vi "AutoCAD cmds testing.vi"(6 "AutoCAD cmd":T3, 7 "MathCAD results":T2, 8 "error in (no error)":errorcluster, 9 "path":path=path "C:/Documents and Settings/mw24/My Documents/Drawing2.dwg", 10 "Command":string="box 4 4 4\n_-view\n_swiso\n_shademode\nRealistic ") -> (0 "error out":errorcluster, 2 "IsQuiescent":bool)   [LabVIEW 2010]
uses:
  AutoCAD cmds.ctl
  MathCAD results ref.ctl
  Project commands.ctl
  AguaClara Library.lvlib
panel:
  in  "AcSaveAsType":T1(ring)
  out "new doc error":errorcluster
  out "Iterations":i32
  out "Visible":bool
  out "appended path":path
  out "basepath":string
  # "acR14_dwg\n AutoCAD R14 DWG (*.dwg)\n \nac2000_dwg\n AutoCAD 2000 DWG (*.dwg)\n \nac2000_dxf\n AutoCAD 2000 DXF (*.dxf)\n \nac2000_Template\n AutoCAD 2000 Drawing Template File (*.dwt)\n \nac2004_dwg\n AutoCAD 2004 DWG (*.dwg)\n \nac2004_dxf\n AutoCAD 2004 DXF (*.dxf)\n \nac2004_Template\n AutoCAD 2004 Drawing Template File (*.dwt)\n \nac2007_dwg\n AutoCAD 2007 DWG (*.dwg)\n \nac2007_dxf\n AutoCAD 2007 DXF (*.dxf)\n \nac2007_Template\n AutoCAD 2007 Drawing Template File (*.dwt)\n \nacNative\n A synonym for the latest drawing release. In this release, this value equals ac2007_dwg."
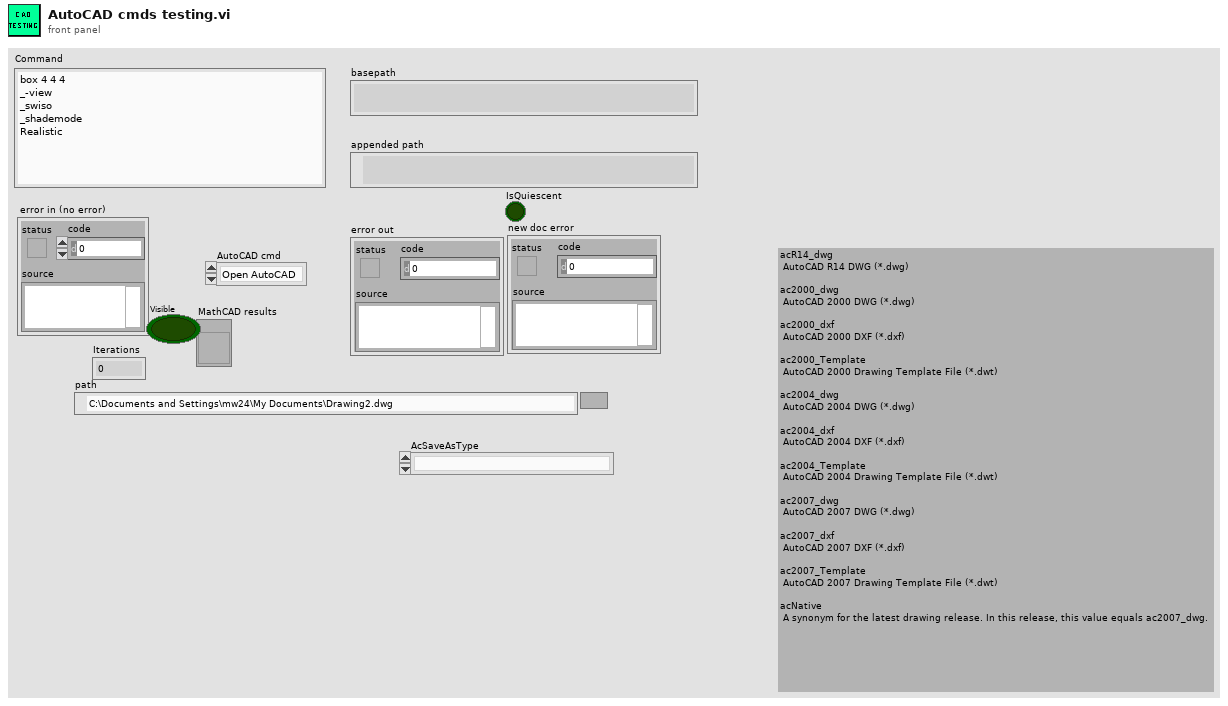
[diagram p1: front panel]
types:
  T1 = enum16{"", "acR14_dwg", "ac2000_dwg", "ac2000_dxf", "ac2000_Template", "ac2004_dwg", "ac2004_dxf", "ac2004_Template", "ac2007_dwg", "ac2007_dxf", "ac2007_Template", "acNative"}
  T2 = typedef "MathCAD results ref.ctl" = refnum<vi>
  T3 = typedef "AguaClara Library.lvlib/AutoCAD cmds.ctl" = enum16{"Open AutoCAD", "New Document", "Send Command", "Send Command Array", "Save picture", "Save File", "Close Doc", "Quit"}
  T4 = typedef "AguaClara Library.lvlib/Project commands.ctl" = enum16{"Load base file", "Load User", "Read paths", "Open Project", "New project", "Edit project", "Delete project", "Mail project", "save design", "open design"}
  T5 = cluster{"Label.Text":string, "Caption.Text":string[], "Control Type":u32, "Numeric":dbl, "Array":dbl[], "status":bool, "Outputs":bool[], "Str Array":string[], "String":string}[]
  T6 = typedef "AguaClara Library.lvlib/File paths.ctl" = cluster{"basepath":string, "AutoCAD script":string, "Design variables":string}
  T7 = typedef "AguaClara Library.lvlib/Project inputs.ctl" = cluster{"Project Name":string, "City":string, "State":string, "Country":string, "Notes":string}
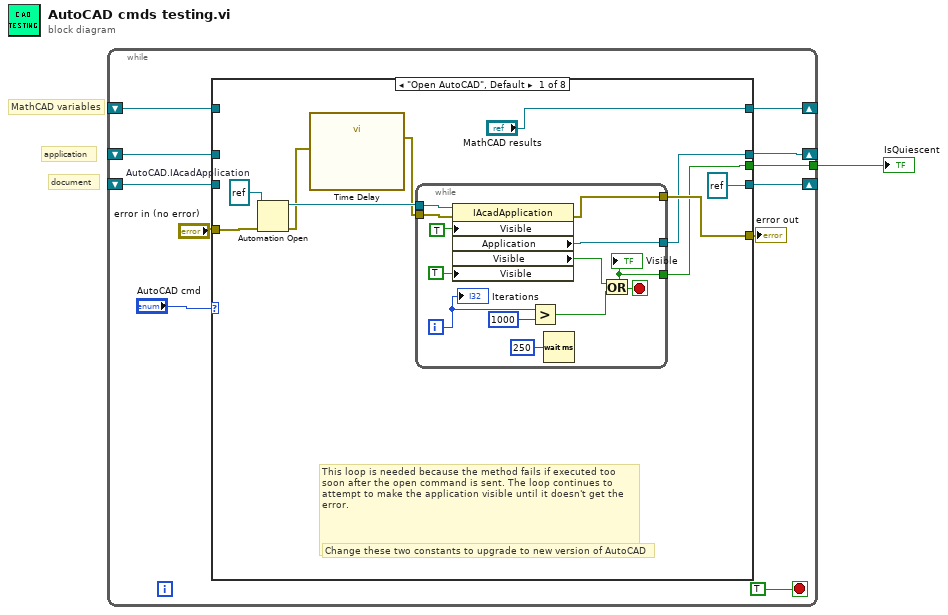
[diagram p0: block diagram]
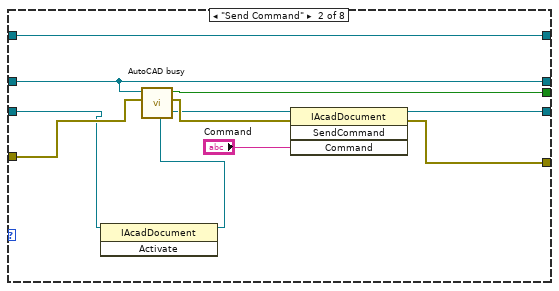
[diagram p2: hidden frame]
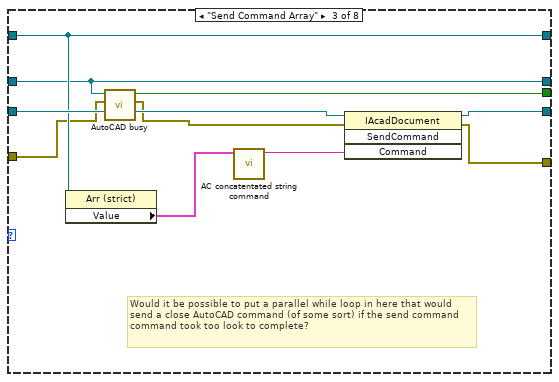
[diagram p3: hidden frame]
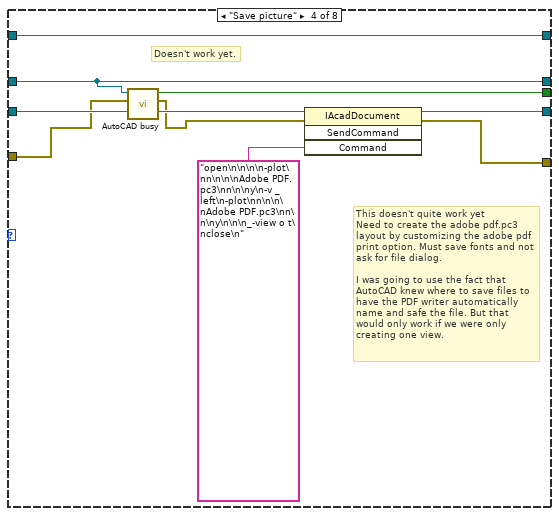
[diagram p4: hidden frame]
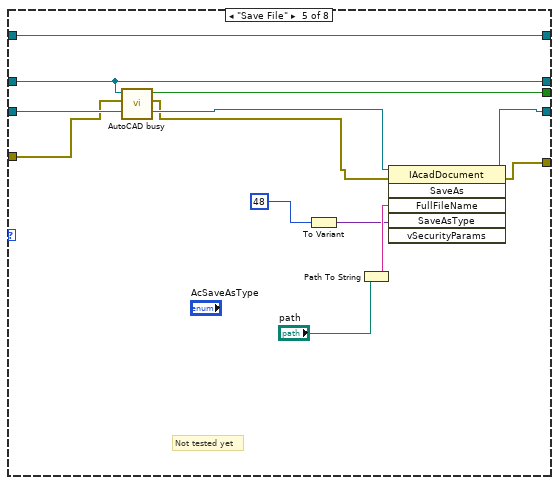
[diagram p5: hidden frame]
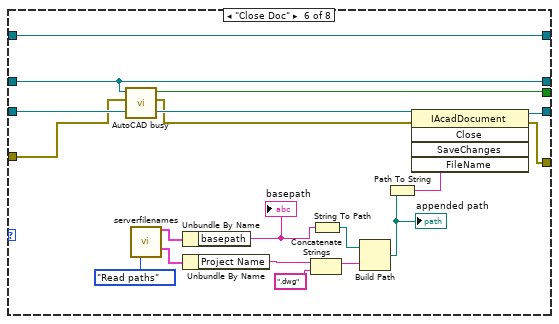
[diagram p6: hidden frame]
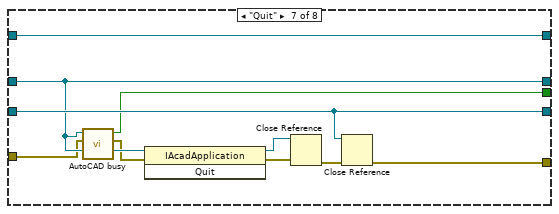
[diagram p7: hidden frame]
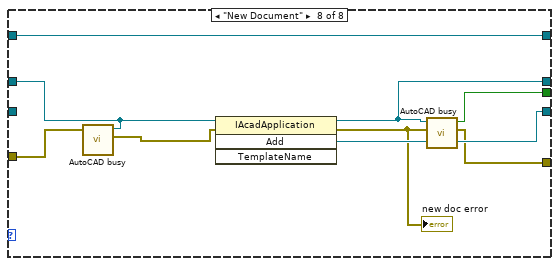
[diagram p8: hidden frame]
diagram:
  # "MathCAD variables"
  # "document"
  # "application"
  n1 = while {
    shift-right: [w11] -> _
    shift-left: _ -> [w6]
    shift-right: [w8] -> _
    shift-left: _ -> [w7]
    shift-right: [w4] -> _
    shift-left: _ -> [w3]
    tunnel: [w2] -> w1
    stop <- TRUE stop-if-true
    n2 = case shown="\"Open AutoCAD\", Default" "AutoCAD cmd" {
      tunnel: [w17 w40 w48 w58 w71 w79 w97 w108] -> w11
      tunnel: "error in (no error)" -> [w13 w39 w47 w57 w70 w78 w96 w109]
      tunnel: [w18 w42 w52 w62 w74 w91 w98 w107] -> w9
      tunnel: [refnum<k7> refnum ("Add") w43 w53 w60 w72 w92 w99 w112] -> w8
      tunnel: w7 -> [_ w36 w54 w61 w73 w93 w99 _]
      tunnel: w6 -> [_ w40 w48 w58 w71 w79 w97 w110]
      tunnel: ["MathCAD results" w41 w51 w63 w75 w80 w103 w111] -> w4
      tunnel: w3 -> [_ w41 w51 w63 w75 w80 w103 w111]
      tunnel: [w16 w37 w45 w55 w68 w76 w94 w106] -> w2
      frame "Open AutoCAD", Default {
        w20 = refnum<k7> refnum  # AutoCAD.IAcadApplication
        # "This loop is needed because the method fails if executed too soon after the open command is sent. The loop continues to attempt to make the application visible until it doesn't get the error."
        # "Change these two constants to upgrade to new version of AutoCAD"
        n3 = Automation Open(error in (no error)=w13, Automation Refnum=w20) -> (Automation Refnum=w19:refnum<k7>, error out=w15:errorcluster)  [unwired: 2 in]
        n4 = call "Time Delay"("error in (no error)"=w15) -> ("error out"=w14:errorcluster)  [unwired: 10 in]
        n5 = while {
          tunnel: w19 -> [w34]
          tunnel: w14 -> [w33]
          tunnel: [w28] -> w18
          tunnel: [w27] -> w17
          tunnel: [w24] -> w16
          i -> [w31]
          stop <- w32 stop-if-true
          n6 = property class="IAcadApplication"(reference=w34, error in=w33, "Visible"=TRUE, "Visible"=TRUE) -> (error out=w28:errorcluster, "Application"=w27:refnum<k7>, "Visible"=w24:bool)  [unwired: 1 out]
          "Visible" <- w24
          n7 = Greater?(x=w31, y=1000) -> (0:w29:bool)
          n8 = Wait (ms)(milliseconds to wait=u32 250) -> ()  [unwired: 1 out]
          n9 = Or(x=w24, y=w29) -> (x .or. y?=w32:bool)
          "Iterations" <- w31
        }
      }
      frame "Send Command" {
        n10 = invoke class="IAcadDocument" method="Activate"(reference=w36) -> (reference out=w35:refnum<k7>)  [unwired: 2 in, 2 out]
        n11 = call "AutoCAD busy.vi"("error in (no error)"=w39, "Application"=w40) -> ("error out"=w38:errorcluster, "IsQuiescent"=w37:bool)  [unwired: 4 in]
        n12 = invoke class="IAcadDocument" method="SendCommand"(reference=w35, error in=w38, "Command"="Command") -> (reference out=w43:refnum<k7>, error out=w42:errorcluster)  [unwired: 1 in, 2 out]
      }
      frame "Send Command Array" {
        # "Would it be possible to put a parallel while loop in here that would send a close AutoCAD command (of some sort) if the send command command took too look to complete?"
        n13 = property class="Arr (strict)"(reference=w51) -> ("Value"=w50:T5)  [unwired: 1 in, 2 out]
        n14 = call "AutoCAD busy.vi"("error in (no error)"=w47, "Application"=w48) -> ("error out"=w46:errorcluster, "IsQuiescent"=w45:bool)  [unwired: 4 in]
        n15 = call "AC concatentated string command.vi"("MathCAD results"=w50) -> ("AC concatenated string"=w49:string)  [unwired: 9 in, 1 out]
        n16 = invoke class="IAcadDocument" method="SendCommand"(reference=w54, error in=w46, "Command"=w49) -> (reference out=w53:refnum<k7>, error out=w52:errorcluster)  [unwired: 1 in, 2 out]
      }
      frame "Save picture" {
        # "Doesn't work yet."
        # "This doesn't quite work yet\nNeed to create the adobe pdf.pc3 layout by customizing the adobe pdf print option. Must save fonts and not ask for file dialog.\n\nI was going to use the fact that AutoCAD knew where to save files to have the PDF writer automatically name and safe the file. But that would only work if we were only creating one view."
        n17 = call "AutoCAD busy.vi"("error in (no error)"=w57, "Application"=w58) -> ("error out"=w56:errorcluster, "IsQuiescent"=w55:bool)  [unwired: 4 in]
        n18 = invoke class="IAcadDocument" method="SendCommand"(reference=w61, error in=w56, "Command"="open\n\n\n\n-plot\nn\n\n\nAdobe PDF.pc3\nn\n\ny\n-v _left\n-plot\nn\n\n\nAdobe PDF.pc3\nn\n\ny\n\n\n_-view o t\nclose\n") -> (reference out=w60:refnum<k7>, error out=w62:errorcluster)  [unwired: 1 in, 2 out]
      }
      frame "Save File" {
        # "Not tested yet"
        n19 = call "AutoCAD busy.vi"("error in (no error)"=w70, "Application"=w71) -> ("error out"=w69:errorcluster, "IsQuiescent"=w68:bool)  [unwired: 4 in]
        n20 = To Variant(anything=i8 48) -> (Variant=w64:variant)
        n21 = Path To String(path="path") -> (string=w65:string)
        n22 = invoke class="IAcadDocument" method="SaveAs"(reference=w73, error in=w69, "FullFileName"=w65, "SaveAsType"=w64) -> (reference out=w72:refnum<k7>, error out=w74:errorcluster)  [unwired: 2 in, 4 out]
      }
      frame "Close Doc" {
        n23 = call "AutoCAD busy.vi"("error in (no error)"=w78, "Application"=w79) -> ("error out"=w77:errorcluster, "IsQuiescent"=w76:bool)  [unwired: 4 in]
        n24 = call "serverfilenames.vi"("Project command"=Project_commands."Read paths") -> ("File paths"=w88:T6, "Project Info out"=w89:T7)  [unwired: 10 in, 3 out]
        n25 = Unbundle By Name(w88) -> ("basepath"=w86:string)
        "basepath" <- w86
        n26 = Unbundle By Name(w89) -> ("Project Name"=w90:string)
        n27 = Concatenate Strings(w90, ".dwg" ("string")) -> (w82:string)
        n28 = String To Path(string=w86) -> (path=w85:path)
        n29 = Build Path(base path=w85, name or relative path=w82) -> (appended path=w84:path)
        "appended path" <- w84
        n30 = Path To String(path=w84) -> (string=w83:string)
        n31 = invoke class="IAcadDocument" method="Close"(reference=w93, error in=w77, "FileName"=w83) -> (reference out=w92:refnum<k7>, error out=w91:errorcluster)  [unwired: 2 in, 3 out]
      }
      frame "Quit" {
        n32 = call "AutoCAD busy.vi"("error in (no error)"=w96, "Application"=w97) -> ("error out"=w95:errorcluster, "IsQuiescent"=w94:bool)  [unwired: 4 in]
        n33 = invoke class="IAcadApplication" method="Quit"(reference=w97, error in=w95) -> (reference out=w102:refnum<k7>, error out=w101:errorcluster)  [unwired: 1 in, 1 out]
        n34 = Close Reference(reference=w102, error in (no error)=w101) -> (error out=w100:errorcluster)
        n35 = Close Reference(reference=w99, error in (no error)=w100) -> (error out=w98:errorcluster)
      }
      frame "New Document" {
        n36 = call "AutoCAD busy.vi"("error in (no error)"=w109, "Application"=w110) -> ("error out"=w104:errorcluster)  [unwired: 4 in, 1 out]
        n37 = invoke class="IAcadApplication" method="Add"(reference=w110, error in=w104) -> (reference out=w108:refnum<k7>, error out=w105:errorcluster, "Add"=w112:refnum<k7>)  [unwired: 2 in, 1 out]
        "new doc error" <- w105
        n38 = call "AutoCAD busy.vi"("error in (no error)"=w105, "Application"=w108) -> ("error out"=w107:errorcluster, "IsQuiescent"=w106:bool)  [unwired: 4 in]
      }
    }
    "error out" <- w9
  }
  "IsQuiescent" <- w1
